vi "Ograniczenie zadanej predkości.vi"(4 "omega [rad/s]":dbl) -> (1 "Wart. ogr.":dbl)   [LabVIEW 2015, in "Biblioteka moduł map v3.lvlib" / "Pomocnicze.lvlib"]
doc: "Ograniczenie minimalnych wartości prędkości kątowych co do wartości bezwzlędnej, gdyż poniżej pewnej wartości koła się nie kręcą."
uses:
  Pomocnicze.lvlib
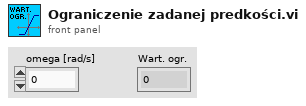
[diagram p1: front panel]
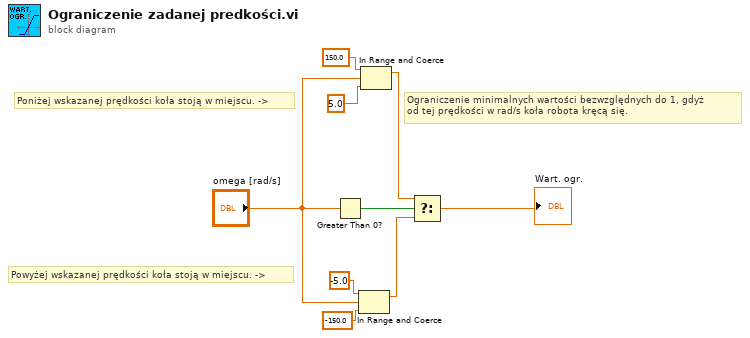
[diagram p0: block diagram]
diagram:
  # "Ograniczenie minimalnych wartości bezwzględnych do 1, gdyż \nod tej prędkości w rad/s koła robota kręcą się."
  # "Powyżej wskazanej prędkości koła stoją w miejscu. ->"
  # "Poniżej wskazanej prędkości koła stoją w miejscu. ->"
  n1 = Greater Than 0?(x="omega [rad/s]") -> (x > 0?=w2:bool)
  n2 = In Range and Coerce(upper limit=-5.0, x="omega [rad/s]", lower limit=-150.0) -> (coerced(x)=w4:dbl)  [unwired: 1 out]
  n3 = In Range and Coerce(upper limit=150.0, x="omega [rad/s]", lower limit=5.0) -> (coerced(x)=w9:dbl)  [unwired: 1 out]
  n4 = Select(t=w9, s=w2, f=w4) -> (s? t:f=→"Wart. ogr.":dbl)
